vi "VariantFacade.vi"(0 "Data In":T6, 2 "Display State In":T2, 3 "Container State":T5) -> (6 "Data Out":T6, 7 "Display State Out":T2, 8 "Action":T1)   [LabVIEW 2013, in "VariantXControl__VP.xctl"]
uses:
  VariantXControl__VP.xctl
  VariantData.ctl
  <vilib>/_xctls/Container State.ctl
  VariantState.ctl
  Permissions.ctl
  TreeSettings.ctl
  <vilib>/_xctls/Action.ctl
  <userlib>/_OpenG.lib/comparison/comparison.llb/Variant Changed__ogtk.vi
  <vilib>/_xctls/XControlSupport.lvlib
panel:
  in  "VariantTree":string(tree)
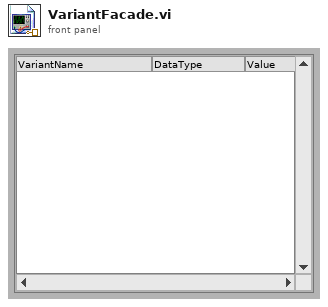
[diagram p1: front panel]
types:
  T1 = typedef "XControlSupport.lvlib/Action.ctl" = cluster{"Data Changed?":bool, "State Changed?":bool, "Action Name":string}
  T2 = typedef "VariantXControl__VP.xctl/VariantState.ctl" = cluster{"State":string, "Messages":cluster{"Message":string, "Parameter":variant}[], "Current run":i32, "Start run":i32, "LastTag":string, "Tags":string[], "Length":i32, "Permissions":T3, "IsProbe?":bool, "Changed":bool, "TreeSettings":T4, "Tree Ref":refnum<vi>}
  T3 = typedef "VariantXControl__VP.xctl/Permissions.ctl" = cluster{"Reset":bool, "TraverseAttributes":bool, "Colorize":bool}
  T4 = typedef "VariantXControl__VP.xctl/TreeSettings.ctl" = cluster{"Traverse":bool, "Colorize":bool}
  T5 = typedef "XControlSupport.lvlib/Container State.ctl" = cluster{"Indicator?":bool, "Run Mode?":bool, " Refnum":refnum<vi>}
  T6 = typedef "VariantXControl__VP.xctl/VariantData.ctl" = variant
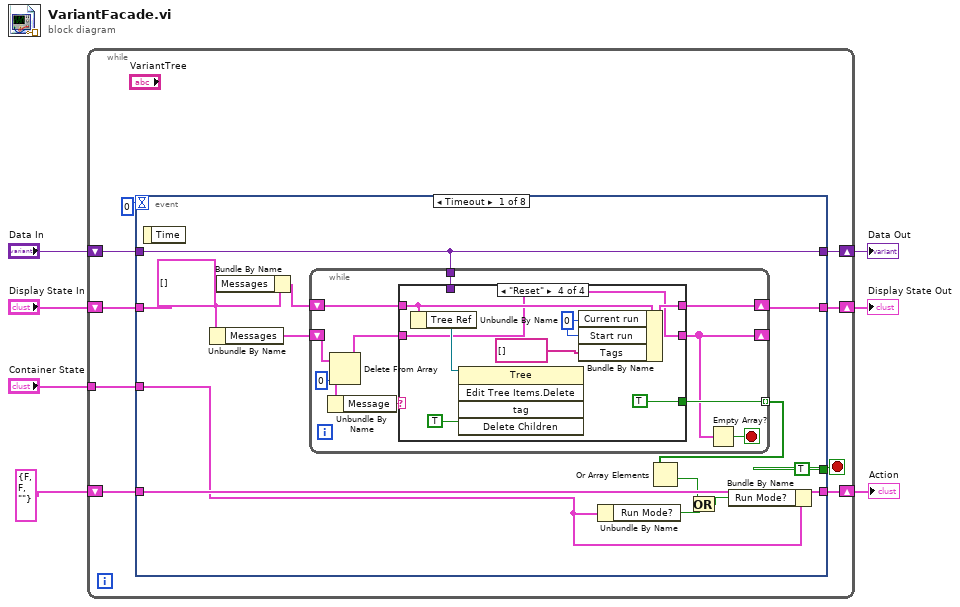
[diagram p0: block diagram]
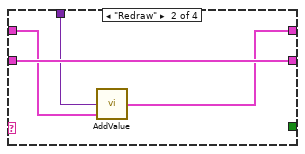
[diagram p3: hidden frame]
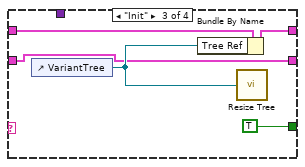
[diagram p4: hidden frame]
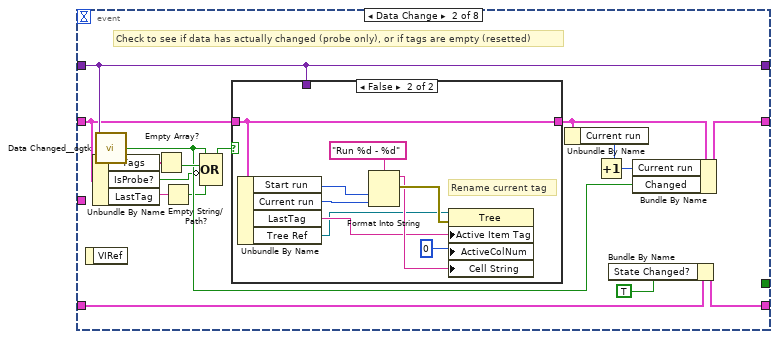
[diagram p5: hidden frame]
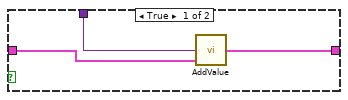
[diagram p6: hidden frame]
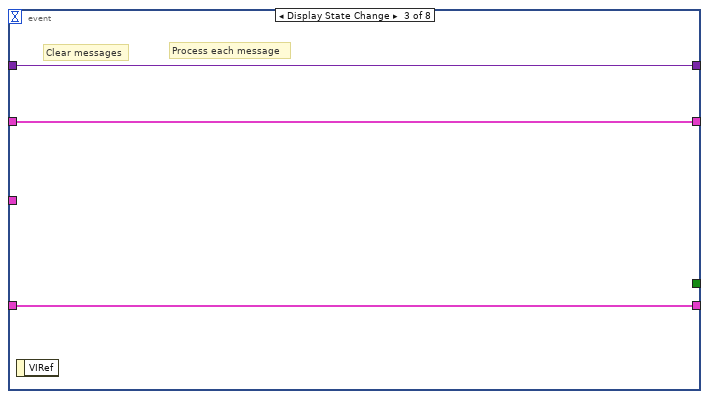
[diagram p7: hidden frame]
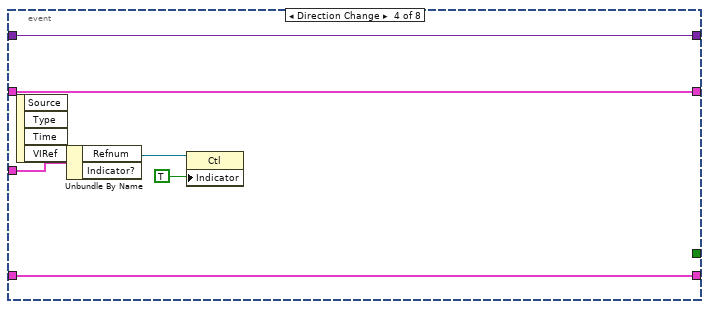
[diagram p8: hidden frame]
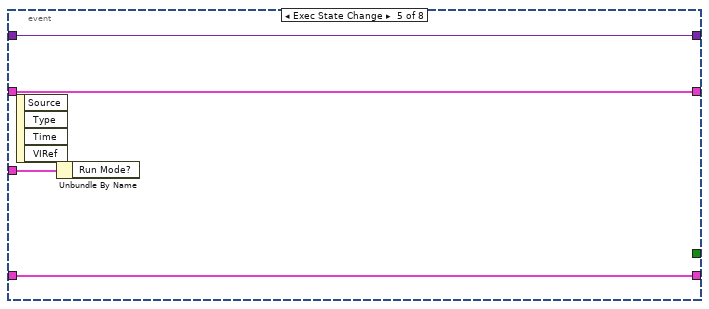
[diagram p9: hidden frame]
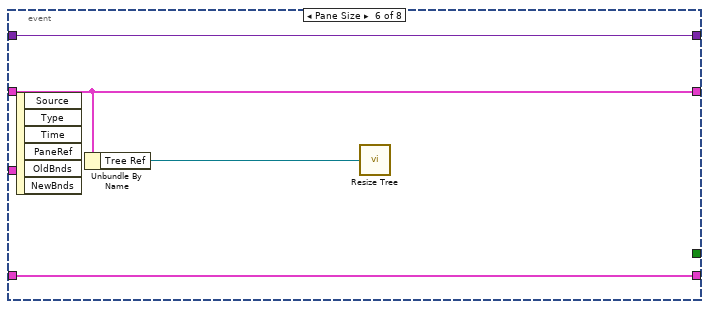
[diagram p10: hidden frame]
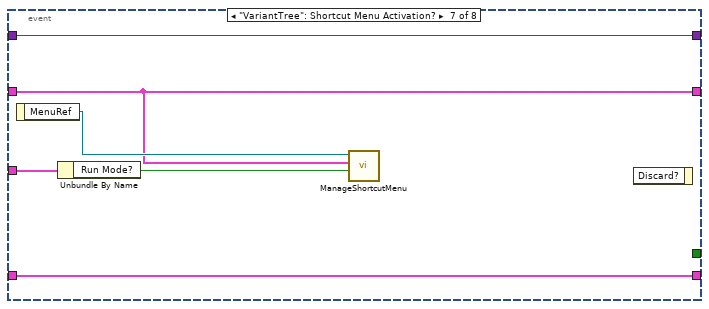
[diagram p11: hidden frame]
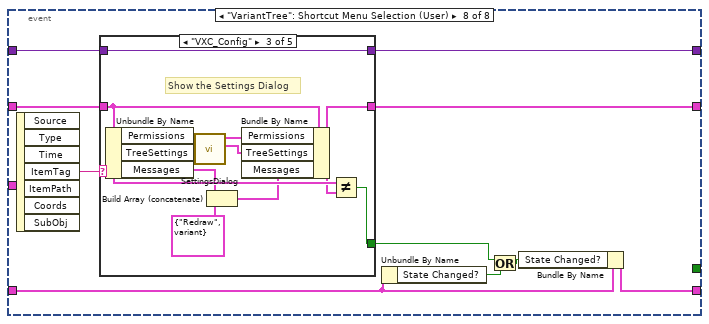
[diagram p12: hidden frame]
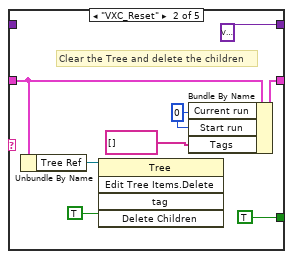
[diagram p14: hidden frame]
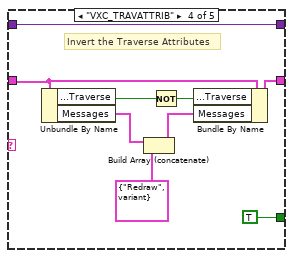
[diagram p15: hidden frame]
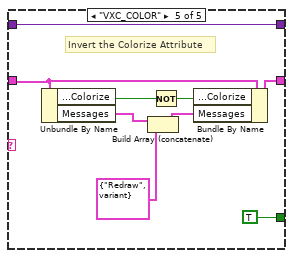
[diagram p16: hidden frame]
diagram:
  n1 = while {
    shift-right: [w15] -> w4
    shift-left: "Display State In" -> [w16]
    tunnel: "Container State" -> [w12]
    shift-right: [w10] -> w7
    shift-left: "Data In" -> [w11]
    shift-right: [w8] -> w2
    shift-left: T1 {"Data Changed?"=FALSE, "State Changed?"=FALSE, "Action Name"=""} ("Action") -> [w9]
    stop <- w14 stop-if-true
    n2 = event shown="[0] Timeout" {
      selector: _ -> [_ _ _ _ _ _ _ _]
      dyn-events: _ -> [_ _ _ _ _ _ _ _]
      timeout: 0 -> [_ _ _ _ _ _ _ _]
      tunnel: w16 -> [w20 w68 w89 w95 w99 w102 w105 w118]
      tunnel: [w18 w71 w89 w95 w99 w102 w105 w117] -> w15
      tunnel: [TRUE _ _ _ _ _ _ _] -> w14
      tunnel: w12 -> [w19 _ _ w96 w100 _ w108 _]
      tunnel: w11 -> [w17 w69 w90 w94 w98 w104 w110 w112]
      tunnel: [w17 w69 w90 w94 w98 w104 w110 w111] -> w10
      tunnel: [w28 w74 w88 w93 w97 w103 w109 w119] -> w8
      tunnel: w9 -> [w28 w75 w88 w93 w97 w103 w109 w116]
      event Timeout {
        n3 = event-data() -> ()  [unwired: 1 in, 1 out]
        n4 = Unbundle By Name(w20) -> ("Messages"=w27:cluster{"Message":string, "Parameter":variant}[])
        n5 = Bundle By Name(cluster=w20, "Messages"=cluster{"Message":string, "Parameter":variant}[] []) -> (w25:T2)
        n6 = while {
          shift-right: [w38] -> w18
          shift-left: w25 -> [w39]
          tunnel: [w37] -> w26 mode=indexing
          shift-right: [w32] -> _
          shift-left: w27 -> [w36]
          tunnel: w17 -> [w30]
          stop <- w31 stop-if-true
          n7 = Delete From Array(array=w36, index=0) -> (deleted portion=w34:cluster{"Message":string, "Parameter":variant}, array with subset deleted=w33:cluster{"Message":string, "Parameter":variant}[])  [unwired: 1 in]
          n8 = Unbundle By Name(w34) -> ("Message"=w40:string)
          n9 = case shown="\"Reset\"" w40 {
            tunnel: w39 -> [w42 w44 w49 w56]
            tunnel: [w42 w43 w51 w59] -> w38
            tunnel: [_ _ TRUE TRUE] -> w37
            tunnel: w33 -> [w41 w46 w47 w52]
            tunnel: [w41 w46 w47 w52] -> w32
            tunnel: w30 -> [_ w45 _ _]
            frame Default {
            }
            frame "Redraw" {
              n10 = call "AddValue.vi"("Display State In"=w44, "Data In"=w45) -> ("Display State Out"=w43:T2)  [unwired: 1 in]
            }
            frame "Init" {
              n11 = control-ref of="VariantTree"() -> (w48:refnum<vi>)
              n12 = Bundle By Name(cluster=w49, "Tree Ref"=w48) -> (w51:T2)
              n13 = call "Resize Tree.vi"("Tree Ref"=w48) -> ()
            }
            frame "Reset" {
              w58 = 0 ("Current run")
              n14 = Unbundle By Name(w56) -> ("Tree Ref"=w53:refnum<vi>)
              n15 = invoke class="Tree" method="Edit Tree Items.Delete"(reference=w53, "Delete Children"=TRUE ("Delete Children?")) -> ()  [unwired: 3 in, 5 out]
              n16 = Bundle By Name(cluster=w56, "Current run"=w58, "Start run"=w58, "Tags"=string[] []) -> (w59:T2)
            }
          }
          n17 = Empty Array?(array=w32) -> (empty?=w31:bool)
        }
        n18 = Unbundle By Name(w19) -> ("Run Mode?"=w23:bool)
        n19 = Or Array Elements(Boolean array=w26) -> (logical OR=w21:bool)
        n20 = Or(x=w21, y=w23) -> (x .or. y?=w22:bool)
        n21 = Bundle By Name(cluster=w19, "Run Mode?"=w22) -> ()  [unwired: 1 out]
      }
      event Data Change {
        # "Check to see if data has actually changed (probe only), or if tags are empty (resetted)"
        n22 = event-data() -> ()  [unwired: 1 in, 1 out]
        n23 = Unbundle By Name(w68) -> ("Tags"=w67:string[], "IsProbe?"=w61:bool, "LastTag"=w63:string)
        n24 = call-poly <userlib>:"Data Changed__ogtk.vi"("Variant"=w69) -> ("Changed"=w64:bool)
        n25 = Empty Array?(array=w67) -> (empty?=w66:bool)
        n26 = Empty String/Path?(string/path=w63) -> (empty?=w62:bool)
        n27 = Compound Arithmetic op=OR(w64, w66, invert w61, w62) -> (w65:bool)
        n28 = case shown="False" w65 {
          tunnel: w68 -> [w78 w80]
          tunnel: w69 -> [w77 _]
          tunnel: [w76 w80] -> w60
          frame True {
            n29 = call "AddValue.vi"("Display State In"=w78, "Data In"=w77) -> ("Display State Out"=w76:T2)  [unwired: 1 in]
          }
          frame False {
            # "Rename current tag"
            n30 = Unbundle By Name(w80) -> ("Start run"=w84:i32, "Current run"=w81:i32, "LastTag"=w82:string, "Tree Ref"=w79:refnum<vi>)
            n31 = Format Into String(format string="Run %d - %d" ("Left Cell String"), w84, w81) -> (resulting string=w85:string, error out=w87:errorcluster)  [unwired: 2 in]
            n32 = property class="Tree"(reference=w79, error in=w87, "Active Item Tag"=w82, "ActiveColNum"=0 ("Active Cell:Active Column Number"), "Cell String"=w85) -> ()  [unwired: 2 out]
          }
        }
        n33 = Unbundle By Name(w60) -> ("Current run"=w70:i32)
        n34 = Increment(x=w70) -> (x+1=w72:i32)
        n35 = Bundle By Name(cluster=w75, "State Changed?"=TRUE) -> (w74:T1)
        n36 = Bundle By Name(cluster=w60, "Current run"=w72, "Changed"=w64) -> (w71:T2)
      }
      event Display State Change {
        # "Process each message"
        # "Clear messages"
        n37 = event-data() -> ()  [unwired: 1 in, 1 out]
      }
      event Direction Change {
        n38 = event-data() -> ()  [unwired: 1 in, 4 out]
        n39 = Unbundle By Name(w96) -> ("Refnum"=w92:refnum<vi>)  [unwired: 1 out]
        n40 = property class="Ctl"(reference=w92, "Indicator"=TRUE) -> ()  [unwired: 1 in, 2 out]
      }
      event Exec State Change {
        n41 = event-data() -> ()  [unwired: 1 in, 4 out]
        n42 = Unbundle By Name(w100) -> ()  [unwired: 1 out]
      }
      event Pane Size {
        n43 = event-data() -> ()  [unwired: 1 in, 6 out]
        n44 = Unbundle By Name(w102) -> ("Tree Ref"=w101:refnum<vi>)
        n45 = call "Resize Tree.vi"("Tree Ref"=w101) -> ()
      }
      event "VariantTree": Shortcut Menu Activation? {
        n46 = event-data() -> ("MenuRef"=w106:refnum<k9>)  [unwired: 1 in]
        n47 = Unbundle By Name(w108) -> ("Run Mode?"=w107:bool)
        n48 = call "ManageShortcutMenu.vi"("Run Mode?"=w107, "Display State In"=w105, "MenuRef"=w106) -> ()  [unwired: 9 in]
        n49 = event-data() -> ()  [unwired: 2 in, 1 out]
      }
      event "VariantTree": Shortcut Menu Selection (User) {
        n50 = event-data() -> ("ItemTag"=w120:string)  [unwired: 1 in, 6 out]
        n51 = case shown="\"VXC_Config\"" w120 {
          tunnel: [_ TRUE w136 TRUE TRUE] -> w115
          tunnel: w118 -> [w122 w127 w135 w148 w157]
          tunnel: [w122 w126 w134 w147 w156] -> w117
          tunnel: w112 -> [w121 _ w139 w150 w159]
          tunnel: [w121 T6 variant ("Data In") w139 w150 w159] -> w111
          frame Default {
          }
          frame "VXC_Reset" {
            w130 = 0 ("Current run")
            # "Clear the Tree and delete the children"
            n52 = Unbundle By Name(w127) -> ("Tree Ref"=w123:refnum<vi>)
            n53 = invoke class="Tree" method="Edit Tree Items.Delete"(reference=w123, "Delete Children"=TRUE ("Delete Children?")) -> ()  [unwired: 3 in, 5 out]
            n54 = Bundle By Name(cluster=w127, "Current run"=w130, "Start run"=w130, "Tags"=string[] []) -> (w126:T2)
          }
          frame "VXC_Config" {
            # "Show the Settings Dialog"
            n55 = Unbundle By Name(w135) -> ("Permissions"=w140:T3, "TreeSettings"=w138:T4, "Messages"=w132:cluster{"Message":string, "Parameter":variant}[])
            n56 = call "SettingsDialog.vi"("TreeSettings In"=w138, "Settings In"=w140) -> ("TreeSettings Out"=w137:T4, "Settings Out"=w141:T3)  [unwired: 8 in]
            n57 = Build Array (concatenate)(w132, cluster{"Message":string, "Parameter":variant} {"Message"="Redraw", "Parameter"=variant} ("Cluster")) -> (w131:cluster{"Message":string, "Parameter":variant}[])
            n58 = Bundle By Name(cluster=w135, "Permissions"=w141, "TreeSettings"=w137, "Messages"=w131) -> (w134:T2)
            n59 = Not Equal?(x=w135, y=w134) -> (x != y?=w136:bool)
          }
          frame "VXC_TRAVATTRIB" {
            # "Invert the Traverse Attributes"
            n60 = Unbundle By Name(w148) -> ("TreeSettings.Traverse"=w146:bool, "Messages"=w143:cluster{"Message":string, "Parameter":variant}[])
            n61 = Build Array (concatenate)(w143, cluster{"Message":string, "Parameter":variant} {"Message"="Redraw", "Parameter"=variant} ("Cluster")) -> (w142:cluster{"Message":string, "Parameter":variant}[])
            n62 = Not(x=w146) -> (.not. x?=w145:bool)
            n63 = Bundle By Name(cluster=w148, "TreeSettings.Traverse"=w145, "Messages"=w142) -> (w147:T2)
          }
          frame "VXC_COLOR" {
            # "Invert the Colorize Attribute"
            n64 = Unbundle By Name(w157) -> ("TreeSettings.Colorize"=w155:bool, "Messages"=w152:cluster{"Message":string, "Parameter":variant}[])
            n65 = Build Array (concatenate)(w152, cluster{"Message":string, "Parameter":variant} {"Message"="Redraw", "Parameter"=variant} ("Cluster")) -> (w151:cluster{"Message":string, "Parameter":variant}[])
            n66 = Not(x=w155) -> (.not. x?=w154:bool)
            n67 = Bundle By Name(cluster=w157, "TreeSettings.Colorize"=w154, "Messages"=w151) -> (w156:T2)
          }
        }
        n68 = Unbundle By Name(w116) -> ("State Changed?"=w114:bool)
        n69 = Or(x=w115, y=w114) -> (x .or. y?=w113:bool)
        n70 = Bundle By Name(cluster=w116, "State Changed?"=w113) -> (w119:T1)
      }
    }
  }
  "Display State Out" <- w4
  "Data Out" <- w7
  "Action" <- w2
